vi "RunTest.vi"(8 "error in (no error)":errorcluster, 11 "TestCase in":refnum<class "TestCase.lvclass">) -> (0 "error out":errorcluster, 3 "TestCase out":refnum<class "TestCase.lvclass">)   [LabVIEW 2019, in "TestCase.lvlib" / "TestCase.lvclass"]
doc: "Override to run the test and assert its state."
uses:
  TestCase.lvclass
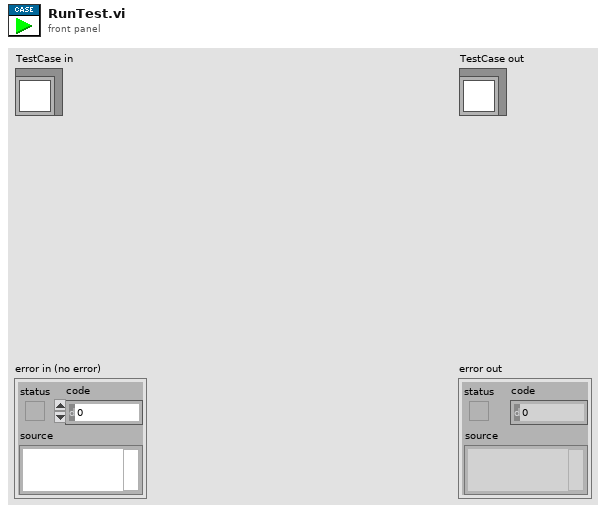
[diagram p1: front panel]
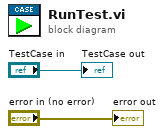
[diagram p0: block diagram]
diagram:
  "error out" <- "error in (no error)"
  "TestCase out" <- "TestCase in"
